vi "Variabile.vi"() -> ()   [LabVIEW 2009]
uses:
  Var_globale.vi
panel:
  in  "Boolean":bool
  in  "Slide":dbl(slide) scale=0.0..10.0
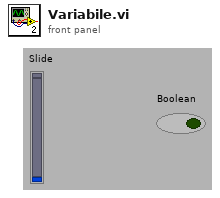
[diagram p1: front panel]
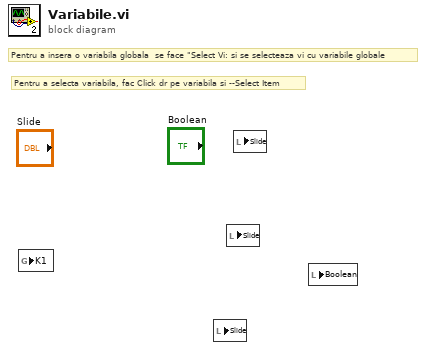
[diagram p0: block diagram]
diagram:
  # "Pentru a selecta variabila, fac Click dr pe variabila si --Select Item"
  # "Pentru a insera o variabila globala  se face \"Select Vi: si se selecteaza vi cu variabile globale"
  n1 = global read "Var_globale.vi" "K1"() -> ()  [unwired: 1 in]
  n2 = local read "Slide"() -> ()  [unwired: 1 in]
  n3 = local read "Slide"() -> ()  [unwired: 1 in]
  n4 = local read "Slide"() -> ()  [unwired: 1 in]
  n5 = local read "Boolean"() -> ()  [unwired: 1 in]
